vi "Read PS Driver.vi"(8 "error in (no error)":errorcluster, 11 "PS Control Persistence Actor in":refnum<class "PS Control Persistence Actor.lvclass">) -> (0 "error out":errorcluster, 2 "PS Driver.lvlib:PS Driver.lvclass":refnum<class "PS Driver.lvclass">, 3 "PS Control Persistence Actor out":refnum<class "PS Control Persistence Actor.lvclass">)   [LabVIEW 2021, in "PS Control Persistence.lvlib" / "PS Control Persistence Actor.lvclass"]
uses:
  PS Control Persistence Actor.lvclass
  PS Driver/PS Driver.lvclass
  PS Control Persistence Actor.lvclass/PS Control Persistence Actor.ctl
  PS Driver/PS Driver with Persistence.lvclass
  Users/Shared/NML Data Acquisition/SCM PS Actor Framework/PS Driver/PS Driver.lvclass
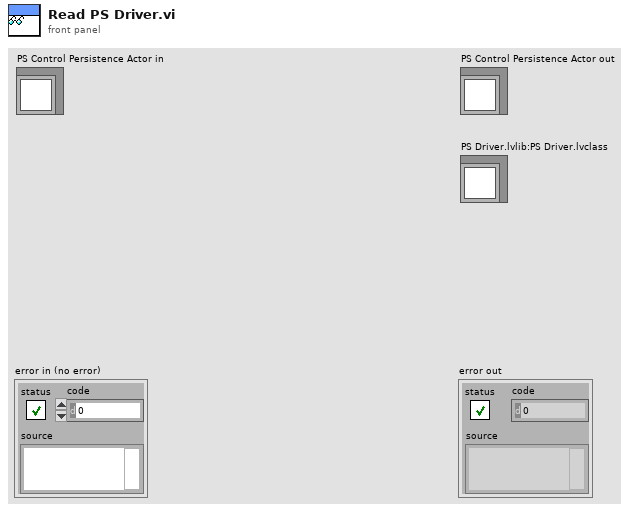
[diagram p1: front panel]
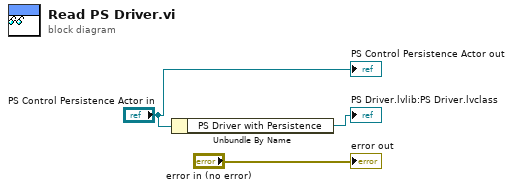
[diagram p0: block diagram]
diagram:
  n1 = Unbundle By Name("PS Control Persistence Actor in") -> ("PS Driver with Persistence"=→"PS Driver.lvlib:PS Driver.lvclass":refnum<class "PS Driver with Persistence.lvclass">)
  "error out" <- "error in (no error)"
  "PS Control Persistence Actor out" <- "PS Control Persistence Actor in"
